vi "setRelaySpec.vi"(1 "Relay Status":bool, 2 "RelaySpec":T1) -> ()   [LabVIEW 2011]
uses:
  relaySpec.ctl
  globals.vi
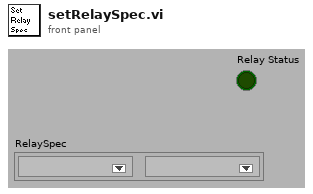
[diagram p1: front panel]
types:
  T1 = typedef "relaySpec.ctl" = cluster{"Card Index":u16, "Relay Index":u16}
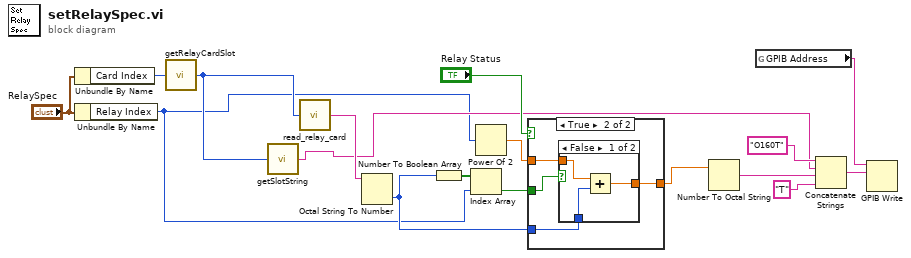
[diagram p0: block diagram]
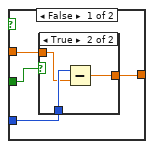
[diagram p2: hidden frame]
diagram:
  n1 = Unbundle By Name("RelaySpec") -> ("Card Index"=w3:u16)
  n2 = Unbundle By Name("RelaySpec") -> ("Relay Index"=w1:u16)
  n3 = call "getRelayCardSlot.vi"("Relay Card Index"=w3) -> ("Slot"=w4:u16)
  n4 = call "getSlotString.vi"("Slot"=w4) -> ("string"=w5:string)
  n5 = call "read_relay_card.vi"("Slot"=w4) -> ("data"=w17:string)
  n6 = Octal String To Number(4:w17) -> (0:w8:u32)  [unwired: 3 out]
  n7 = Number To Boolean Array(number=w8) -> (Boolean array=w13:bool[])
  n8 = Index Array(array=w13, index=w1) -> (element=w12:bool)
  n9 = Power Of 2(x=w1) -> (2^x=w10:dbl)
  n10 = case shown="True" "Relay Status" {
    tunnel: w12 -> [w18 w29]
    tunnel: w8 -> [w19 w28]
    tunnel: w10 -> [w20 w27]
    tunnel: [w21 w26] -> w11
    frame False {
      n11 = case shown="True" w18 {
        tunnel: w19 -> [w22 w24]
        tunnel: w20 -> [_ w23]
        tunnel: [w22 w25] -> w21
        frame False {
        }
        frame True {
          n12 = Subtract(x=w24, y=w23) -> (x-y=w25:dbl)
        }
      }
    }
    frame True {
      n13 = case shown="False" w29 {
        tunnel: w28 -> [w32 w33]
        tunnel: w27 -> [w31 _]
        tunnel: [w30 w33] -> w26
        frame False {
          n14 = Add(x=w31, y=w32) -> (x+y=w30:dbl)
        }
        frame True {
        }
      }
    }
  }
  n15 = Number To Octal String(2:w11) -> (0:w7:string)  [unwired: 1 out]
  n16 = global read "globals.vi" "GPIB Address"() -> (w16:string)
  n17 = Concatenate Strings("O160T", w5, w7, "T" ("string")) -> (w9:string)
  n18 = GPIB Write(0:w16, 1:w9) -> ()  [unwired: 1 in, 4 out]
